vi "Alarm Clock State Machine.vi"() -> ()   [LabVIEW 2013]
panel:
  in  "Stop Alarm":bool
  out "Alarm Indicator":bool
  in  "Set Alarm":bool
  in  "Minute":dbl
  in  "Hour":dbl
  out "Time Dispay":string
  in  "Stop":bool
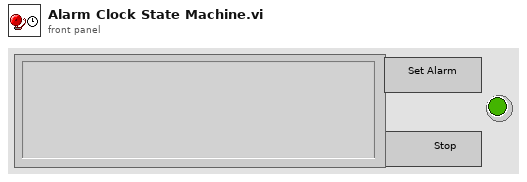
[diagram p1: front panel]
types:
  T1 = enum16{"Display Time", "Set Alarm", "Compare", "Turn Alarm On"}
  T2 = typedef "LVDateTimeRec.ctl" = cluster{"fractional second":dbl, "second":i32, "minute":i32, "hour":i32, "day of month":i32, "month":i32, "year":i32, "day of week":i32, "day of year":i32, "DST":i32}
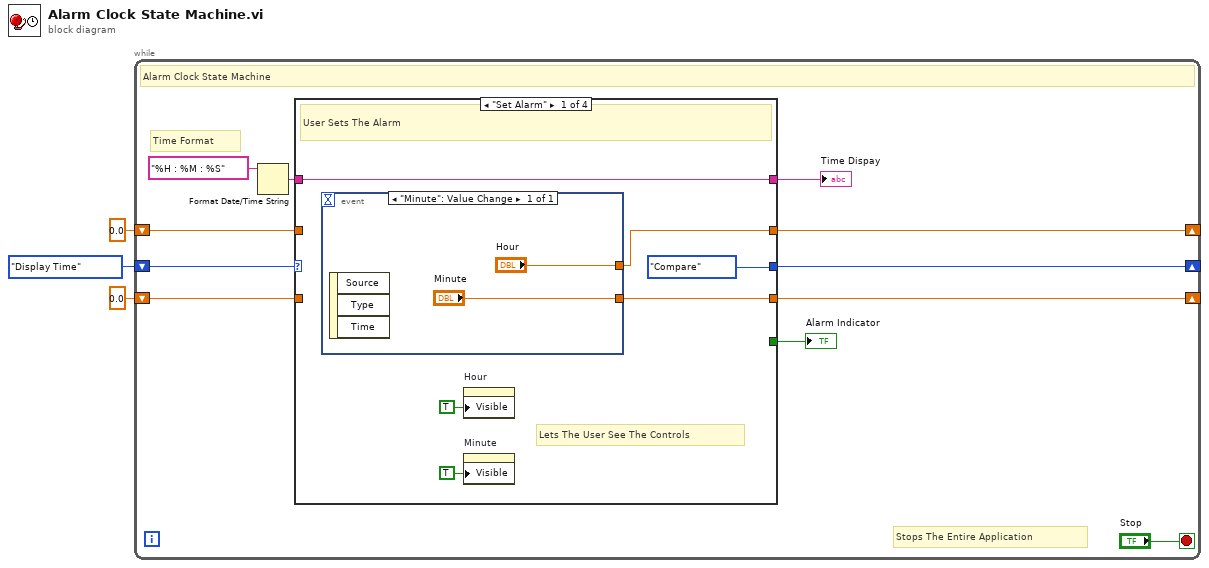
[diagram p0: block diagram]
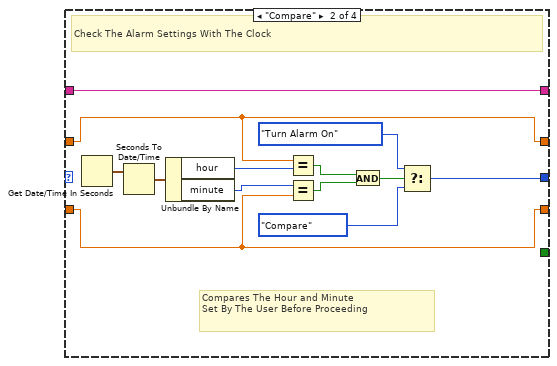
[diagram p2: hidden frame]
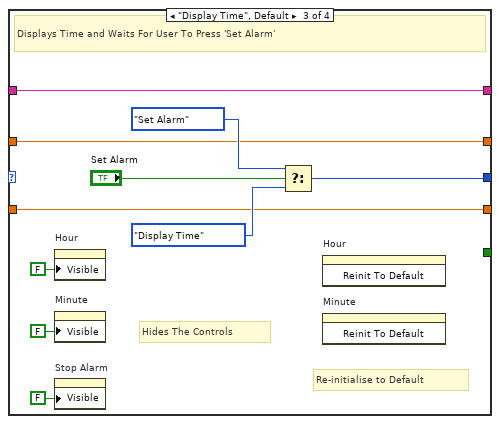
[diagram p3: hidden frame]
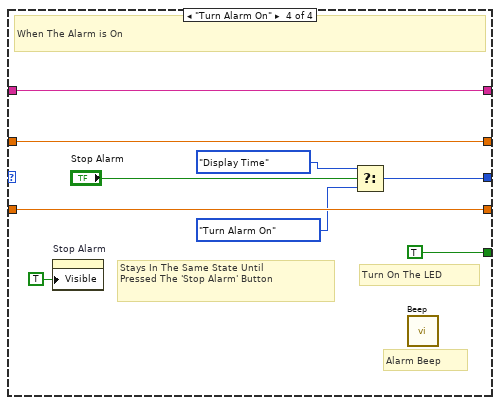
[diagram p4: hidden frame]
diagram:
  n1 = while {
    shift-right: [w10] -> _
    shift-left: T1."Display Time" -> [w14]
    shift-right: [w9] -> _
    shift-left: 0.0 ("Hour") -> [w7]
    shift-right: [w8] -> _
    shift-left: 0.0 ("Minute") -> [w6]
    stop <- "Stop" stop-if-true
    # "Stops The Entire Application"
    # "Time Format"
    # "Alarm Clock State Machine"
    n2 = Format Date/Time String(time format string (%c)="%H : %M : %S") -> (date/time string=w11:string)  [unwired: 2 in]
    n3 = case shown="\"Set Alarm\"" w14 {
      tunnel: [w20 w35 w45 w54] -> w13
      tunnel: w11 -> [w20 w35 w45 w54]
      tunnel: [T1."Compare" w27 w39 w50] -> w10
      tunnel: [w17 w25 w41 w53] -> w9
      tunnel: [w16 w23 w40 w52] -> w8
      tunnel: w7 -> [_ w25 w41 w53]
      tunnel: w6 -> [_ w23 w40 w52]
      tunnel: [_ _ _ TRUE] -> w4
      frame "Set Alarm" {
        # "Lets The User See The Controls"
        # "User Sets The Alarm"
        n4 = event shown="[0] \"Minute\": Value Change" {
          selector: _ -> [_]
          dyn-events: _ -> [_]
          timeout: _ -> [_]
          tunnel: ["Hour"] -> w17
          tunnel: ["Minute"] -> w16
          event "Minute": Value Change {
            n5 = event-data() -> ()  [unwired: 1 in, 3 out]
          }
        }
        n6 = property on="Hour" class="DigNum (strict)"("Visible"=TRUE) -> ()  [unwired: 2 in, 2 out]
        n7 = property on="Minute" class="DigNum (strict)"("Visible"=TRUE) -> ()  [unwired: 2 in, 2 out]
      }
      frame "Compare" {
        # "Compares The Hour and Minute\nSet By The User Before Proceeding"
        # "Check The Alarm Settings With The Clock"
        n8 = Get Date/Time In Seconds() -> (seconds since 1Jan1904=w33:timestamp)
        n9 = Seconds To Date/Time(time stamp (now)=w33) -> (date time rec=w34:T2)  [unwired: 1 in]
        n10 = Unbundle By Name(w34) -> ("hour"=w26:i32, "minute"=w24:i32)
        n11 = Equal?(x=w25, y=w26) -> (x = y?=w32:bool)
        n12 = Equal?(x=w24, y=w23) -> (x = y?=w31:bool)
        n13 = And(x=w32, y=w31) -> (x .and. y?=w30:bool)
        n14 = Select(t=T1."Turn Alarm On", s=w30, f=T1."Compare") -> (s? t:f=w27:T1)
      }
      frame "Display Time", Default {
        # "Re-initialise to Default"
        # "Hides The Controls"
        # "Displays Time and Waits For User To Press 'Set Alarm'"
        n15 = property on="Hour" class="DigNum (strict)"("Visible"=FALSE) -> ()  [unwired: 2 in, 2 out]
        n16 = property on="Minute" class="DigNum (strict)"("Visible"=FALSE) -> ()  [unwired: 2 in, 2 out]
        n17 = property on="Stop Alarm" class="Bool"("Visible"=FALSE) -> ()  [unwired: 2 in, 2 out]
        n18 = Select(t=enum16{"Display Time", "Set Alarm", "Compare"}."Set Alarm", s="Set Alarm", f=enum16{"Display Time", "Set Alarm", "Compare"}."Display Time") -> (s? t:f=w39:enum16{"Display Time", "Set Alarm", "Compare"})
        n19 = invoke on="Hour" class="DigNum (strict)" method="Reinit To Default"() -> ()  [unwired: 3 in, 3 out]
        n20 = invoke on="Minute" class="DigNum (strict)" method="Reinit To Default"() -> ()  [unwired: 3 in, 3 out]
      }
      frame "Turn Alarm On" {
        # "Turn On The LED"
        # "Alarm Beep"
        # "Stays In The Same State Until\nPressed The 'Stop Alarm' Button"
        # "When The Alarm is On"
        n21 = property on="Stop Alarm" class="Bool"("Visible"=TRUE) -> ()  [unwired: 2 in, 2 out]
        n22 = Select(t=T1."Display Time", s="Stop Alarm", f=T1."Turn Alarm On") -> (s? t:f=w50:T1)
        n23 = call <vilib>:"Beep.vi"() -> ()  [unwired: 12 in]
      }
    }
    "Time Dispay" <- w13
    "Alarm Indicator" <- w4
  }
